vi "Get Joystick Values.vi"(8 "error in (no error)":errorcluster, 11 "Two Drivers in":refnum<class "Two Drivers.lvclass">) -> (0 "error out":errorcluster, 2 "Joystick Data":T1, 3 "Two Drivers out":refnum<class "Two Drivers.lvclass">)   [LabVIEW 2018, in "Joysticks.lvlib" / "Two Drivers.lvclass"]
doc: "Use this method to get the joystick values in a cluster you can use for your application.\n\nModify the Type Def that this VI resturns to fit the controls needed for the robot."
uses:
  Two Drivers.lvclass
  C:/Users/Public/Documents/2019DeepSpace/Classes/Joysticks/Joysticks.lvclass
  Controls/JoystickData.ctl
  Two Drivers.lvclass/Two Drivers.ctl
  Joysticks.lvclass/Joysticks.ctl
  Public Methods/Read Sensitivity(x).vi
  Public Methods/Read Sensitivity(y).vi
  <vilib>/Rock Robotics/WPI/Utilities/WPI_GetSetVariantRefNum.vi
  Private Methods/POV Conditioning.vi
  Joysticks.lvclass
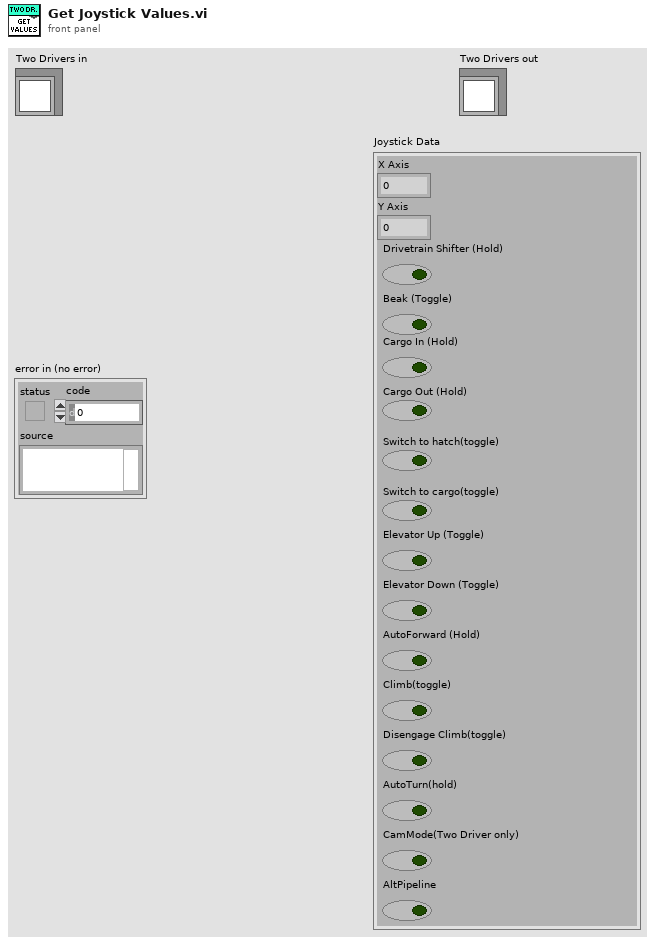
[diagram p1: front panel]
types:
  T1 = typedef "Joysticks.lvlib/Joysticks.lvclass/JoystickData.ctl" = cluster{"X Axis":dbl, "Y Axis":dbl, "Drivetrain Shifter (Hold)":bool, "Beak (Toggle)":bool, "Cargo In (Hold)":bool, "Cargo Out (Hold)":bool, "Switch to hatch(toggle)":bool, "Switch to cargo(toggle)":bool, "Elevator Up (Toggle)":bool, "Elevator Down (Toggle)":bool, "AutoForward (Hold)":bool, "Climb(toggle)":bool, "Disengage Climb(toggle)":bool, "AutoTurn(hold)":bool, "CamMode(Two Driver only)":bool, "AltPipeline":bool}
  T2 = typedef "WPI_JoystickDevRef.ctl" = cluster{"Device":T3}
  T3 = typedef "WPI_JoystickDeviceEnum.ctl" = enum16{"USB 0", "USB 1", "USB 2", "USB 3", "USB 4", "USB 5"}
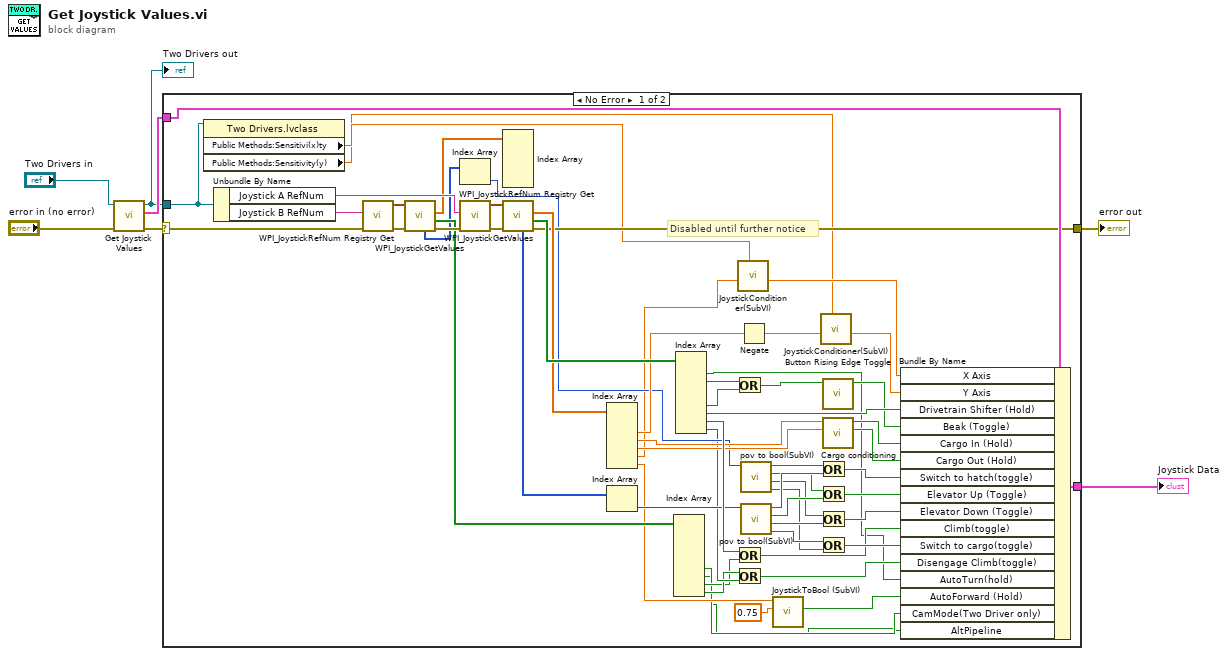
[diagram p0: block diagram]
diagram:
  n1 = call-parent "Get Joystick Values.vi"("error in (no error)"="error in (no error)", "Joysticks in"="Two Drivers in") -> ("error out"=w3:errorcluster, "Joystick Data"=w5:T1, "Joysticks out"=w1:refnum<class "Two Drivers.lvclass">)  [unwired: 7 in]
  "Two Drivers out" <- w1
  n2 = case shown="No Error" w3 {
    selector: w3 -> [w58 w68]
    tunnel: [w51 w68] -> w6
    tunnel: w1 -> [w24 _]
    tunnel: [w64 _] -> w7
    tunnel: w5 -> [w52 _]
    frame No Error {
      # "Disabled until further notice"
      n3 = property class="Two Drivers.lvclass"(reference=w24) -> ("Public Methods:Sensitivi(x)ty"=w23:dbl, "Public Methods:Sensitivity(y)"=w22:dbl)  [unwired: 1 in, 2 out]
      n4 = Unbundle By Name(w24) -> ("Joystick A RefNum"=w66:string, "Joystick B RefNum"=w55:string)
      n5 = call <vilib>:"WPI_JoystickRefNum Registry Get.vi"("error in (no error)"=w58, "refnum name"=w55) -> ("error out"=w57:errorcluster, "JoystickDevRef"=w59:T2)  [unwired: 8 in]
      n6 = call <vilib>:"WPI_JoystickGetValues.vi"("error in (no error)"=w57, "JoystickDevRef"=w59) -> ("error out"=w56:errorcluster, "Buttons"=w53:bool[], "Axes"=w54:dbl[], "POVs"=w37:i16[])  [unwired: 5 in, 1 out]
      n7 = Index Array(array=w37) -> (element=w38:i16)  [unwired: 1 in]
      n8 = call <vilib>:"WPI_JoystickRefNum Registry Get.vi"("error in (no error)"=w56, "refnum name"=w66) -> ("error out"=w67:errorcluster, "JoystickDevRef"=w65:T2)  [unwired: 8 in]
      n9 = Index Array(array=w54) -> ()  [unwired: 5 in, 5 out]
      n10 = call <vilib>:"WPI_JoystickGetValues.vi"("error in (no error)"=w67, "JoystickDevRef"=w65) -> ("error out"=w51:errorcluster, "Buttons"=w63:bool[], "Axes"=w62:dbl[], "POVs"=w50:i16[])  [unwired: 5 in, 1 out]
      n11 = Index Array(array=w62) -> (element #2=w60:dbl, element #3=w43:dbl, element #4=w42:dbl, element #5=w26:dbl, element #6=w13:dbl)  [unwired: 6 in, 1 out]
      n12 = Index Array(array=w50) -> (element=w44:i16)  [unwired: 1 in]
      n13 = Index Array(array=w53) -> (element #5=w10:bool, element #6=w9:bool, element #7=w17:bool, element #8=w19:bool)  [unwired: 8 in, 4 out]
      n14 = Index Array(array=w63) -> (element #1=w8:bool, element #2=w16:bool, element #5=w14:bool, element #6=w61:bool, element #7=w45:bool, element #8=w21:bool)  [unwired: 8 in, 2 out]
      n15 = Or(x=w16, y=w14) -> (x .or. y?=w15:bool)
      n16 = Or(x=w45, y=w17) -> (x .or. y?=w18:bool)
      n17 = Or(x=w19, y=w21) -> (x .or. y?=w20:bool)
      n18 = call "JoystickConditioner(SubVI).vi"("Sensitivity"=w23, "joystick axis"=w26) -> ("output"=w25:dbl)  [unwired: 9 in]
      n19 = Negate(x=w60) -> (-x=w28:dbl)
      n20 = call "pov to bool(SubVI).vi"("Numeric"=w38) -> ("Left"=w35:bool, "Down"=w33:bool, "Up"=w31:bool, "Right"=w29:bool)  [unwired: 7 in]
      n21 = call "pov to bool(SubVI).vi"("Numeric"=w44) -> ("Left"=w39:bool, "Down"=w47:bool, "Up"=w48:bool, "Right"=w49:bool)  [unwired: 7 in]
      n22 = call "JoystickToBool (SubVI).vi"("Treshhold"=0.75 ("y"), "Axis"=w13) -> ("AutoForward"=w11:bool)  [unwired: 8 in, 1 out]
      n23 = Or(x=w29, y=w49) -> (x .or. y?=w30:bool)
      n24 = Or(x=w31, y=w48) -> (x .or. y?=w32:bool)
      n25 = Or(x=w33, y=w47) -> (x .or. y?=w34:bool)
      n26 = Or(x=w39, y=w35) -> (x .or. y?=w36:bool)
      n27 = call "JoystickConditioner(SubVI).vi"("Sensitivity"=w22, "joystick axis"=w28) -> ("output"=w27:dbl)  [unwired: 9 in]
      n28 = call "Button Rising Edge Toggle.vi"("Button"=w15) -> ("Rising edge?"=w46:bool)  [unwired: 10 in]
      n29 = call "Cargo conditioning.vi"("Cargo Out (Axis)"=w42, "Cargo In (Axis)"=w43) -> ("Cargo Out (Hold)"=w40:bool, "Cargo In (Hold)"=w41:bool)  [unwired: 8 in]
      n30 = Bundle By Name(cluster=w52, "X Axis"=w25, "Y Axis"=w27, "Drivetrain Shifter (Hold)"=w61, "Beak (Toggle)"=w46, "Cargo In (Hold)"=w41, "Cargo Out (Hold)"=w40, "Switch to hatch(toggle)"=w30, "Elevator Up (Toggle)"=w32, "Elevator Down (Toggle)"=w34, "Climb(toggle)"=w18, "Switch to cargo(toggle)"=w36, "Disengage Climb(toggle)"=w20, "AutoTurn(hold)"=w8, "AutoForward (Hold)"=w11, "CamMode(Two Driver only)"=w10, "AltPipeline"=w9) -> (w64:T1)
    }
    frame Error {
    }
  }
  "error out" <- w6
  "Joystick Data" <- w7
